vi "ConfigDevice.vi"(8 "error in (no error)":errorcluster, 11 "ChromaAcLoad in":refnum<class "ChromaAcLoad.lvclass">) -> (0 "error out":errorcluster, 3 "ChromaAcLoad out":refnum<class "ChromaAcLoad.lvclass">)   [LabVIEW 2018, in "AcPwrPlugins.lvlib" / "ChromaAcLoad.lvclass"]
doc: "This VI configures the instrument based on the INI file settings or changes to these settings made using the PrefDialog.vi."
uses:
  ChromaAcLoad.lvclass
  C:/Users/ico/Documents/Projects/NistPluggableModules/AcPwr/AcPwrPlugins/AcPwrBaseClass/AcPwrBase.lvclass
  AcPwrBaseClass/AcPwrBase.lvclass/AcPwrBase.ctl
  TypeDefs/RangeCheck.ctl
  AcPwrBaseClass/Accessors/Read BaseConfig.vi
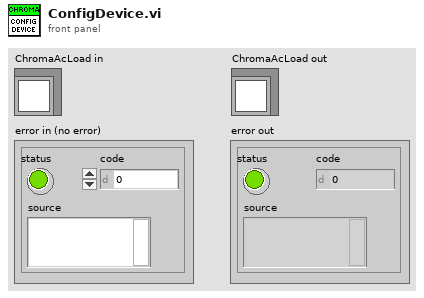
[diagram p1: front panel]
types:
  T1 = typedef "AcPwrPlugins.lvlib/AcPwrBase.lvclass/BaseConfig.ctl" = cluster{"Frequency":dbl, "FrequencyRange":dbl[], "Phases":T2[], "Name":string, "Chroma":T3, "NHRDC":T4, "PPS":T5}
  T2 = typedef "AcPwrPlugins.lvlib/AcPwrBase.lvclass/Phase.ctl" = cluster{"Name":string, "Enabled":bool, "VoltageLevel":dbl, "Handle":string, "VoltageRange":dbl[], "Connected":bool, "CurrentLimit":dbl, "Waveform":string}
  T3 = typedef "AcPwrPlugins.lvlib/ChromaAcLoad.lvclass/DeviceProperties.ctl" = cluster{"Configuration Mode":enum16{"Constant Voltage (DC)", "Constant Power (DC)", "Constant Power (AC)", "Constant Current (DC)", "Constant Current (AC)", "Constant Resistance (DC)", "Constant Resistance (AC)", "Rectified Mode (DC)", "Inrush (AC)", "RLC CP (AC)", "RLC (AC)"}, "Phases":cluster{"Handle":string, "Name":string, "Phase Select":i32, "Instrument Options":string, "id query (T)":bool, "reset device (T)":bool, "Load Short Circuited":bool, "Line Synchronization":bool, "Load Current (A/Arms)":dbl, "Load Voltage (V/Vrms)":dbl, "Load Power (W)":dbl, "Load Resistance (Ohms)":dbl, "Load Current Peak Limit (A)":dbl, "Load Current Limit (A/Arms)":dbl, "Load Power Limit (W)":dbl, "Synch Frequency (Hz)":dbl, "Priority":enum16{"CF Only", "PF Only", "Both (CF)", "Both (PF)"}, "Crest Factor":dbl, "Power Factor":dbl, "Slew Rate":cluster{"Rise Slew Rate (A/ms)":i32, "Fall Slew Rate (A/ms)":i32}, "LC/RLC Mode":cluster{"Capacitance (uF)":i32, "Inductance (uH)":i32, "Series Resistance (Ohm)":dbl, "Parallel Resistance (Ohm)":dbl}, "Timing":cluster{"TimingOn":enum16{""}, "Hours":u32, "Minutes":u32, "Seconds":dbl, "CutoffVoltage":dbl}, "Connected":bool}[]}
  T4 = typedef "AcPwrPlugins.lvlib/NHRDCPower.lvclass/Device(s)Settings.ctl" = cluster{"Handle":string, "Name":string, "id query (Yes)":bool, "reset device (Yes)":bool, "Connected":bool, "Voltage Range (V)":dbl[], "Timing":cluster{"TimingOn":enum16{""}, "Hours":u32, "Minutes":u32, "Seconds":dbl, "CutoffVoltage":dbl}, "Initial Battery Detect Voltage (0)":sgl, "SafetySettings":cluster{"SetWatchDog":bool, "Voltage (V)":sgl, "Current (A)":sgl, "Power (W)":sgl, "Voltage Delay (s)":sgl, "Current Delay (s)":sgl, "Power Delay (s)":sgl}, "Options String":string, "Aperture Time (s)":sgl, "operating state (Off)":i32, "OutputSettings":cluster{"Voltage (V)":sgl, "Current (A)":sgl, "Resistance (Ohms)":sgl, "Power (W)":sgl, "Enable Voltage":bool, "Enable Current":bool, "Enable Resistance":bool, "Enable Power":bool, "Delay After (s)":sgl, "Wait Value (V, A, W)":sgl, "Enable Wait":bool, "Wait on Value":i32}[], "SlewRate":cluster{"Set Voltage Rate V/S":sgl, "Set Current Rate A/S":sgl, "Set Resistance Rate R/S":sgl, "Set Power Rate W/S":sgl}}[]
  T5 = typedef "AcPwrPlugins.lvlib/PacificPowerSource.lvclass/DeviceSettings.ctl" = cluster{"Handle":string, "Connected":bool, "Clear Device (F)":bool, "btnIdQuery":bool, "btnReset":bool, "Program #":cluster{"Phase B (Degrees)":i32, "Waveform A (1: Sine)":i32, "Voltage Level (Va)":dbl, "Program Number (0)":i32, "Voltage Level (Vb) ":dbl, "Form (3: Three)":u16, "Coupling  (0: Direct)":u16, "Frequency (45Hz)":dbl, "Current Limit (40A)":dbl, "Phase C (Degrees)":i32, "Voltage Level (Vc)":dbl, "Waveform B (1: Sine)":i32, "Waveform C (1: Sine)":i32}[], "Impedance Parameters (off, 0.00)":cluster{"State":bool, "Impedance":dbl}, "Transient Execution (F)":bool, "OutputEnabled":bool, "Source Range":cluster{"Frequency Minimum (45 Hz)":dbl, "Frequency Maximum (1200 Hz)":dbl, "Voltage Maximum (V)":dbl, "Voltage Minimum (V)":dbl, "Range Control (0: Auto)":u16, "Initial Voltage (0V)":u16, "Frequency Range (600Hz)":u16}, "Port Type":enum16{"GPIB", "Serial"}}[]
  T6 = enum16{"Constant Voltage (DC)", "Constant Power (DC)", "Constant Power (AC)", "Constant Current (DC)", "Constant Current (AC)", "Constant Resistance (DC)", "Constant Resistance (AC)", "Rectified Mode (DC)", "Inrush (AC)", "RLC CP (AC)", "RLC (AC)"}
  T7 = cluster{"Handle":string, "Name":string, "Phase Select":i32, "Instrument Options":string, "id query (T)":bool, "reset device (T)":bool, "Load Short Circuited":bool, "Line Synchronization":bool, "Load Current (A/Arms)":dbl, "Load Voltage (V/Vrms)":dbl, "Load Power (W)":dbl, "Load Resistance (Ohms)":dbl, "Load Current Peak Limit (A)":dbl, "Load Current Limit (A/Arms)":dbl, "Load Power Limit (W)":dbl, "Synch Frequency (Hz)":dbl, "Priority":enum16{"CF Only", "PF Only", "Both (CF)", "Both (PF)"}, "Crest Factor":dbl, "Power Factor":dbl, "Slew Rate":cluster{"Rise Slew Rate (A/ms)":i32, "Fall Slew Rate (A/ms)":i32}, "LC/RLC Mode":cluster{"Capacitance (uF)":i32, "Inductance (uH)":i32, "Series Resistance (Ohm)":dbl, "Parallel Resistance (Ohm)":dbl}, "Timing":cluster{"TimingOn":enum16{""}, "Hours":u32, "Minutes":u32, "Seconds":dbl, "CutoffVoltage":dbl}, "Connected":bool}[]
  T8 = typedef "AcPwrPlugins.lvlib/ChromaAcLoad.lvclass/RangeCheck.ctl" = enum16{"Power", "Power Limit", "Current", "Current Peak", "Current Limit", "Voltage", "AC Resistance", "DC Resistance", "Frequency", "Crest Factor", "Power Factor", "RLC Power Factor", "Rise Slew Rate", "Fall Slew Rate", "Capacitance", "Inductance", "Parallel Resistance", "Series Resistance"}[]
  T9 = enum16{"CF Only", "PF Only", "Both (CF)", "Both (PF)"}
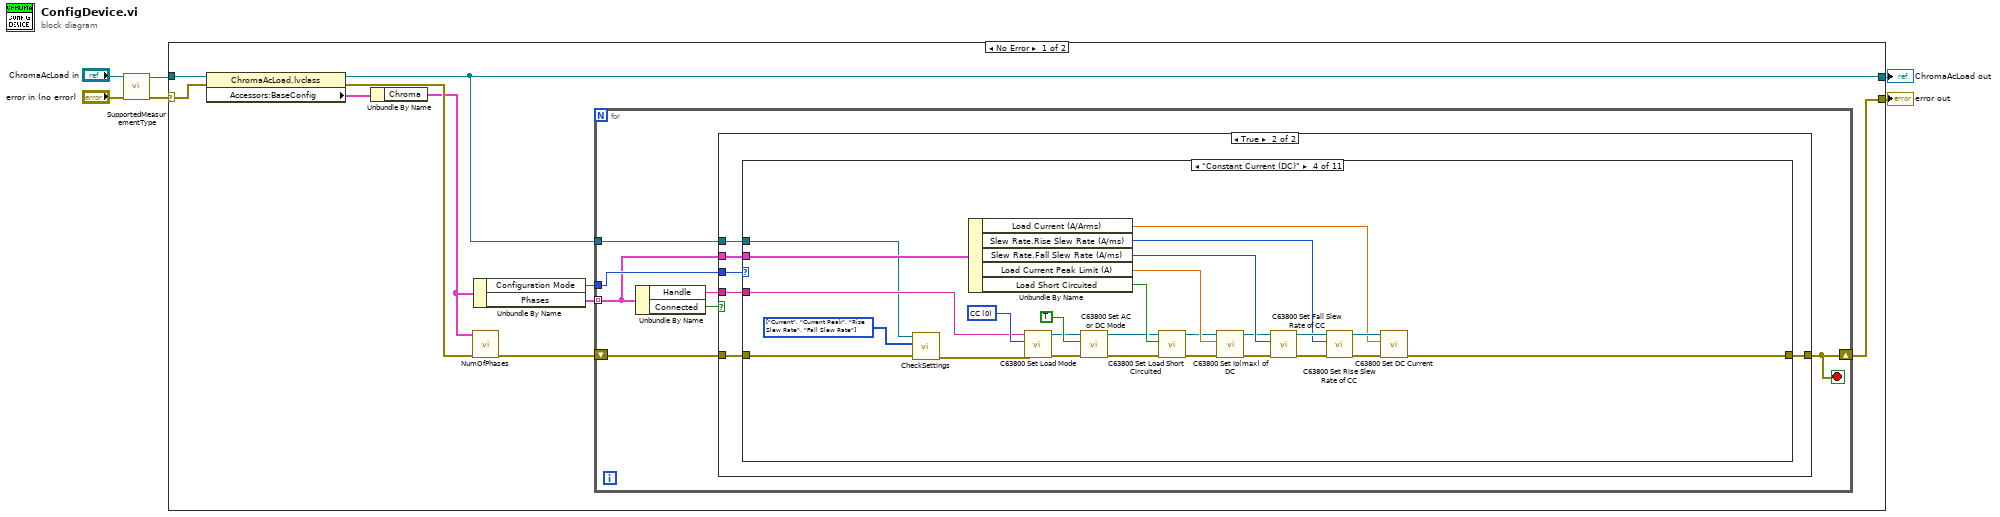
[diagram p0: block diagram]
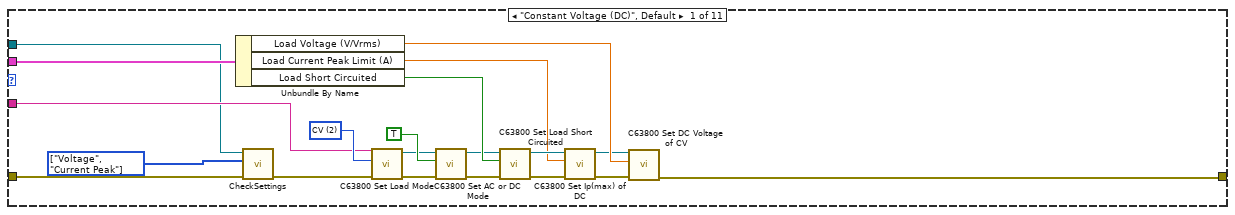
[diagram p3: hidden frame]
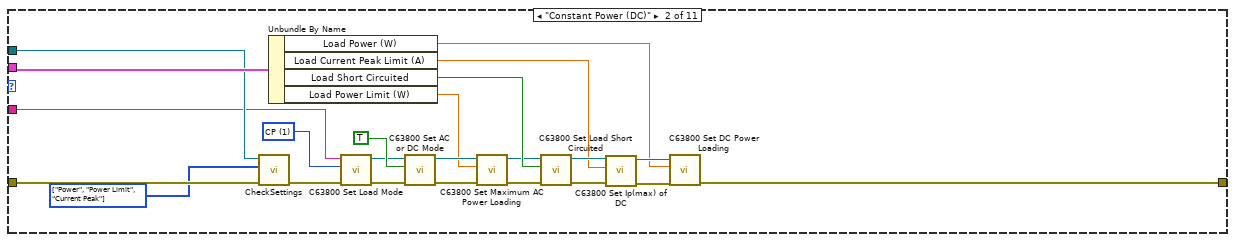
[diagram p4: hidden frame]
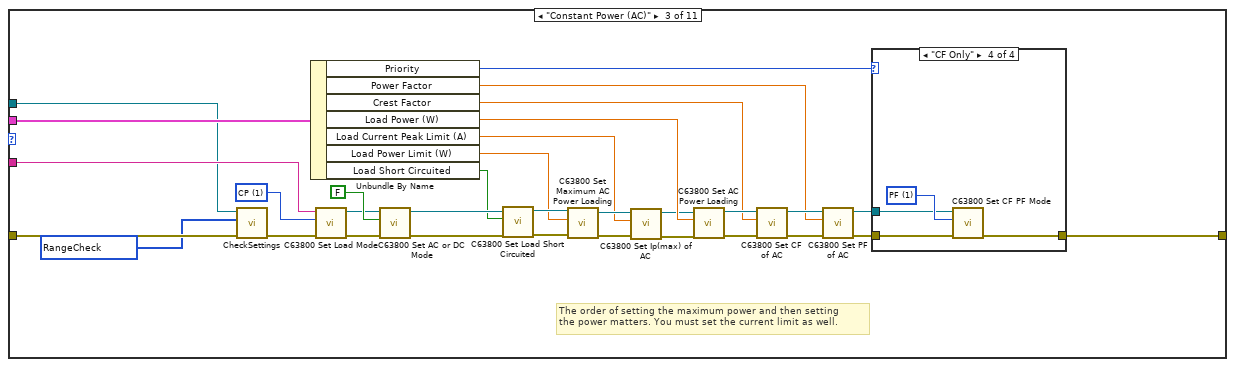
[diagram p5: hidden frame]
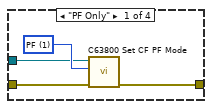
[diagram p6: hidden frame]
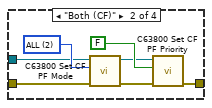
[diagram p7: hidden frame]
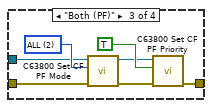
[diagram p8: hidden frame]
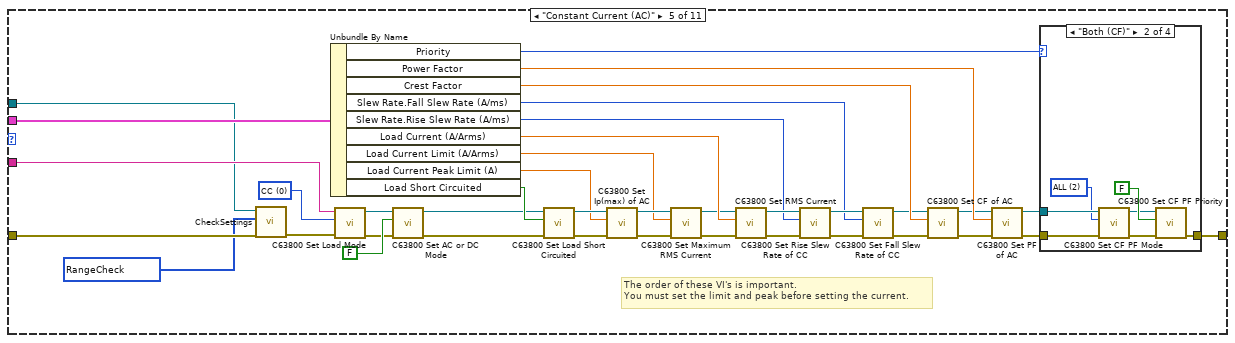
[diagram p9: hidden frame]
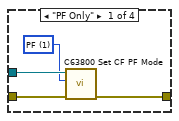
[diagram p10: hidden frame]
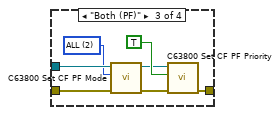
[diagram p11: hidden frame]
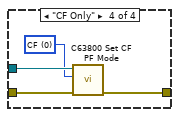
[diagram p12: hidden frame]
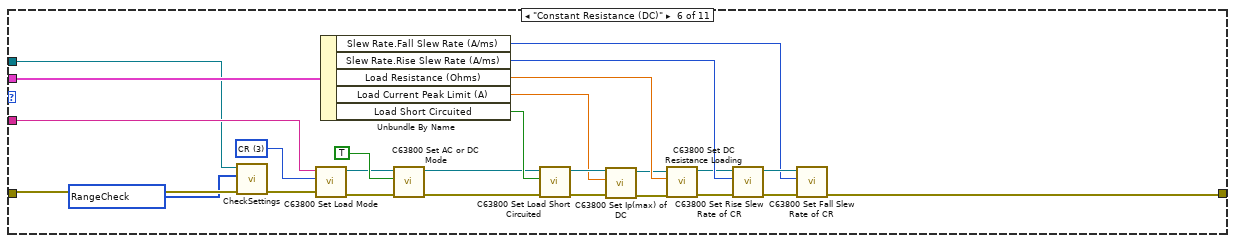
[diagram p13: hidden frame]
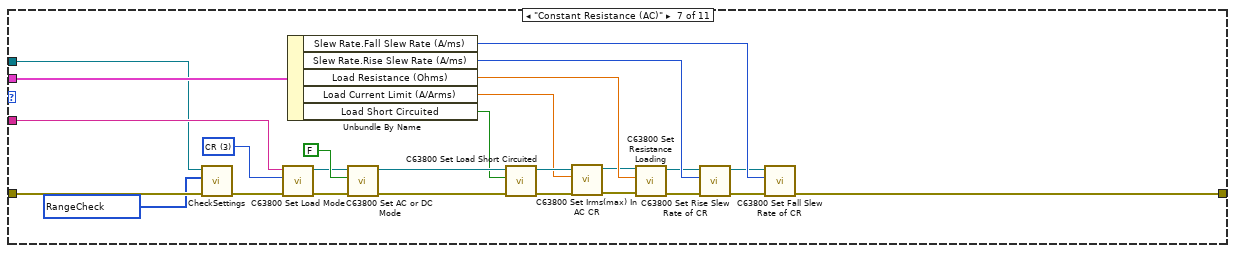
[diagram p14: hidden frame]
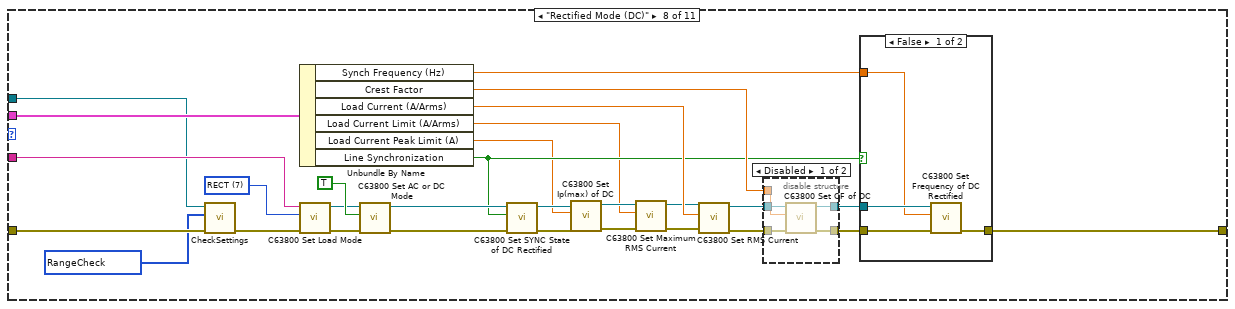
[diagram p15: hidden frame]
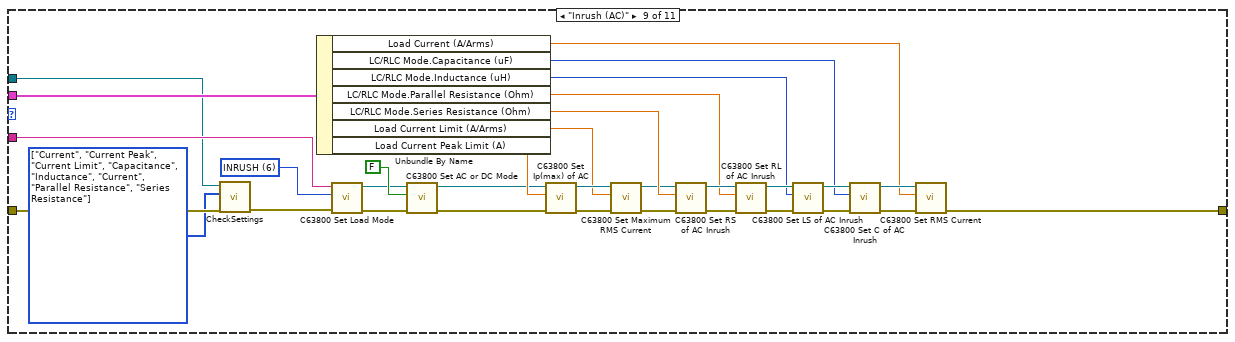
[diagram p18: hidden frame]
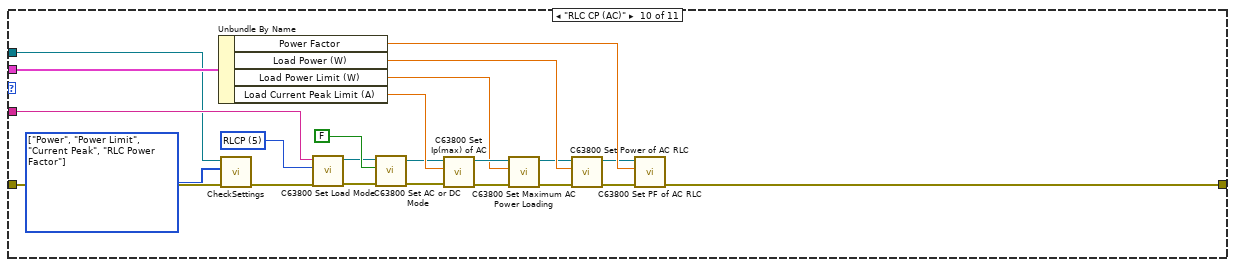
[diagram p19: hidden frame]
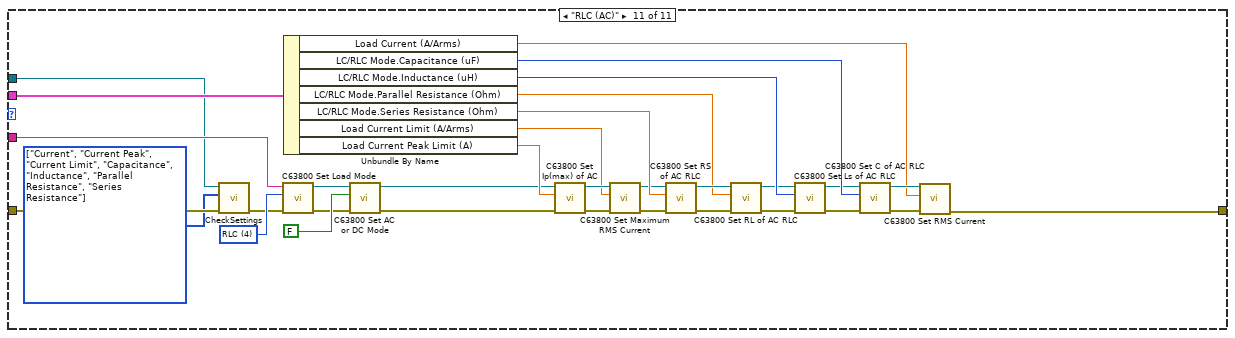
[diagram p20: hidden frame]
diagram:
  n1 = call-dynamic "SupportedMeasurementType.vi"("error in (no error)"="error in (no error)", "ChromaAcLoad in"="ChromaAcLoad in") -> ("error out"=w3:errorcluster, "ChromaAcLoad out"=w4:refnum<class "ChromaAcLoad.lvclass">)  [unwired: 8 in]
  n2 = case shown="No Error" w3 {
    selector: w3 -> [w16 w391]
    tunnel: [w15 w391] -> w6
    tunnel: w4 -> [w14 w390]
    tunnel: [w13 w390] -> w5
    frame No Error {
      n3 = property class="ChromaAcLoad.lvclass"(reference=w14, error in=w16) -> (reference out=w13:refnum<class "ChromaAcLoad.lvclass">, error out=w9:errorcluster, "Accessors:BaseConfig"=w8:T1)
      n4 = Unbundle By Name(w8) -> ("Chroma"=w7:T3)
      n5 = call "NumOfPhases.vi"("Error In"=w9, "Device Properties"=w7) -> ("Error Out"=w10:errorcluster)  [unwired: 8 in, 1 out]
      n6 = Unbundle By Name(w7) -> ("Configuration Mode"=w11:T6, "Phases"=w12:T7)
      n7 = for {
        shift-right: [w20] -> w15
        shift-left: w10 -> [w21]
        tunnel: w12 -> [w18] mode=indexing
        tunnel: w11 -> [w23]
        tunnel: w13 -> [w17]
        stop <- w20 stop-if-true
        n8 = Unbundle By Name(w18) -> ("Handle"=w19:string, "Connected"=w22:bool)
        n9 = case shown="True" w22 {
          tunnel: w23 -> [_ w28]
          tunnel: w21 -> [w24 w30]
          tunnel: [w24 w29] -> w20
          tunnel: w19 -> [_ w27]
          tunnel: w18 -> [_ w26]
          tunnel: w17 -> [_ w25]
          frame False {
          }
          frame True {
            n10 = case shown="\"Constant Current (DC)\"" w28 {
              tunnel: w30 -> [w39 w71 w102 w137 w167 w218 w252 w278 w314 w347 w371]
              tunnel: [w41 w69 w105 w128 w178 w228 w261 w286 w310 w342 w364] -> w29
              tunnel: w27 -> [w43 w70 w103 w140 w173 w221 w255 w279 w316 w349 w373]
              tunnel: w26 -> [w49 w73 w104 w146 w179 w226 w260 w285 w323 w356 w378]
              tunnel: w25 -> [w37 w72 w101 w136 w166 w216 w250 w276 w315 w345 w368]
              frame "Constant Voltage (DC)", Default {
                w36 = T8 [enum."Voltage", enum."Current Peak"] items=["Power", "Power Limit", "Current", "Current Peak", "Current Limit", "Voltage", "AC Resistance", "DC Resistance", "Frequency", "Crest Factor", "Power Factor", "RLC Power Factor", "Rise Slew Rate", "Fall Slew Rate", "Capacitance", "Inductance", "Parallel Resistance", "Series Resistance"] ("RangeCheck")
                w45 = 2 items=["CC", "CP", "CV", "CR", "RLC", "RLCP", "INRUSH", "RECT"] ("Load Mode")
                n11 = Unbundle By Name(w49) -> ("Load Voltage (V/Vrms)"=w40:dbl, "Load Current Peak Limit (A)"=w31:dbl, "Load Short Circuited"=w50:bool)
                n12 = call-dynamic "CheckSettings.vi"("ChromaAcLoad in"=w37, "RangeCheck"=w36, "error in (no error)"=w39) -> ("error out"=w38:errorcluster)  [unwired: 6 in, 1 out]
                n13 = call <instrlib>:"C63800 Set Load Mode.vi"("error in (no error)"=w38, "Load Mode"=w45, "Instrument Handle"=w43) -> ("error out"=w44:errorcluster, "Instrument Handle out"=w42:refnum<k15>)  [unwired: 7 in]
                n14 = call <instrlib>:"C63800 Set AC or DC Mode.vi"("error in (no error)"=w44, "Select AC_DC Mode"=TRUE, "Instrument Handle"=w42) -> ("error out"=w48:errorcluster, "Instrument Handle out"=w46:refnum<k15>)  [unwired: 7 in]
                n15 = call <instrlib>:"C63800 Set Load Short Circuited.vi"("error in (no error)"=w48, "Short Circuited State"=w50, "Instrument Handle"=w46) -> ("error out"=w35:errorcluster, "Instrument Handle out"=w32:refnum<k15>)  [unwired: 7 in]
                n16 = call <instrlib>:"C63800 Set Ip(max) of DC.vi"("error in (no error)"=w35, "I_max_DC"=w31, "Instrument Handle"=w32) -> ("error out"=w33:errorcluster, "Instrument Handle out"=w34:refnum<k15>)  [unwired: 7 in]
                n17 = call <instrlib>:"C63800 Set DC Voltage of CV.vi"("error in (no error)"=w33, "SetDCVoltageofCV"=w40, "Instrument Handle"=w34) -> ("error out"=w41:errorcluster)  [unwired: 7 in, 1 out]
              }
              frame "Constant Power (DC)" {
                w60 = T8 [enum."Power", enum."Power Limit", enum."Current Peak"] items=["Power", "Power Limit", "Current", "Current Peak", "Current Limit", "Voltage", "AC Resistance", "DC Resistance", "Frequency", "Crest Factor", "Power Factor", "RLC Power Factor", "Rise Slew Rate", "Fall Slew Rate", "Capacitance", "Inductance", "Parallel Resistance", "Series Resistance"] ("RangeCheck")
                w66 = 1 items=["CC", "CP", "CV", "CR", "RLC", "RLCP", "INRUSH", "RECT"] ("Load Mode")
                n18 = call-dynamic "CheckSettings.vi"("ChromaAcLoad in"=w72, "RangeCheck"=w60, "error in (no error)"=w71) -> ("error out"=w63:errorcluster)  [unwired: 6 in, 1 out]
                n19 = Unbundle By Name(w73) -> ("Load Power (W)"=w55:dbl, "Load Current Peak Limit (A)"=w54:dbl, "Load Short Circuited"=w68:bool, "Load Power Limit (W)"=w51:dbl)
                n20 = call <instrlib>:"C63800 Set Load Mode.vi"("error in (no error)"=w63, "Load Mode"=w66, "Instrument Handle"=w70) -> ("error out"=w65:errorcluster, "Instrument Handle out"=w64:refnum<k15>)  [unwired: 7 in]
                n21 = call <instrlib>:"C63800 Set AC or DC Mode.vi"("error in (no error)"=w65, "Select AC_DC Mode"=TRUE, "Instrument Handle"=w64) -> ("error out"=w52:errorcluster, "Instrument Handle out"=w53:refnum<k15>)  [unwired: 7 in]
                n22 = call <instrlib>:"C63800 Set Maximum AC Power Loading.vi"("error in (no error)"=w52, "AC Maximum Power Loading"=w51, "Instrument Handle"=w53) -> ("error out"=w62:errorcluster, "Instrument Handle out"=w61:refnum<k15>)  [unwired: 7 in]
                n23 = call <instrlib>:"C63800 Set Load Short Circuited.vi"("error in (no error)"=w62, "Short Circuited State"=w68, "Instrument Handle"=w61) -> ("error out"=w59:errorcluster, "Instrument Handle out"=w56:refnum<k15>)  [unwired: 7 in]
                n24 = call <instrlib>:"C63800 Set Ip(max) of DC.vi"("error in (no error)"=w59, "I_max_DC"=w54, "Instrument Handle"=w56) -> ("error out"=w58:errorcluster, "Instrument Handle out"=w57:refnum<k15>)  [unwired: 7 in]
                n25 = call <instrlib>:"C63800 Set DC Power Loading.vi"("error in (no error)"=w58, "DC Power Loading"=w55, "Instrument Handle"=w57) -> ("error out"=w69:errorcluster)  [unwired: 7 in, 1 out]
              }
              frame "Constant Power (AC)" {
                w93 = T8 [enum."Power", enum."Power Limit", enum."Current Peak", enum."Power Factor", enum."Crest Factor"] items=["Power", "Power Limit", "Current", "Current Peak", "Current Limit", "Voltage", "AC Resistance", "DC Resistance", "Frequency", "Crest Factor", "Power Factor", "RLC Power Factor", "Rise Slew Rate", "Fall Slew Rate", "Capacitance", "Inductance", "Parallel Resistance", "Series Resistance"] ("RangeCheck")
                w97 = 1 items=["CC", "CP", "CV", "CR", "RLC", "RLCP", "INRUSH", "RECT"] ("Load Mode")
                # "The order of setting the maximum power and then setting \nthe power matters. You must set the current limit as well."
                n26 = call-dynamic "CheckSettings.vi"("ChromaAcLoad in"=w101, "RangeCheck"=w93, "error in (no error)"=w102) -> ("error out"=w94:errorcluster)  [unwired: 6 in, 1 out]
                n27 = Unbundle By Name(w104) -> ("Priority"=w90:T9, "Power Factor"=w82:dbl, "Crest Factor"=w83:dbl, "Load Power (W)"=w92:dbl, "Load Current Peak Limit (A)"=w77:dbl, "Load Power Limit (W)"=w74:dbl, "Load Short Circuited"=w91:bool)
                n28 = call <instrlib>:"C63800 Set Load Mode.vi"("error in (no error)"=w94, "Load Mode"=w97, "Instrument Handle"=w103) -> ("error out"=w96:errorcluster, "Instrument Handle out"=w95:refnum<k15>)  [unwired: 7 in]
                n29 = call <instrlib>:"C63800 Set AC or DC Mode.vi"("error in (no error)"=w96, "Select AC_DC Mode"=FALSE, "Instrument Handle"=w95) -> ("error out"=w100:errorcluster, "Instrument Handle out"=w99:refnum<k15>)  [unwired: 7 in]
                n30 = call <instrlib>:"C63800 Set Load Short Circuited.vi"("error in (no error)"=w100, "Short Circuited State"=w91, "Instrument Handle"=w99) -> ("error out"=w75:errorcluster, "Instrument Handle out"=w76:refnum<k15>)  [unwired: 7 in]
                n31 = call <instrlib>:"C63800 Set Maximum AC Power Loading.vi"("error in (no error)"=w75, "AC Maximum Power Loading"=w74, "Instrument Handle"=w76) -> ("error out"=w81:errorcluster, "Instrument Handle out"=w78:refnum<k15>)  [unwired: 7 in]
                n32 = call <instrlib>:"C63800 Set Ip(max) of AC.vi"("error in (no error)"=w81, "Current Peak Max"=w77, "Instrument Handle"=w78) -> ("error out"=w80:errorcluster, "Instrument Handle out"=w79:refnum<k15>)  [unwired: 7 in]
                n33 = call <instrlib>:"C63800 Set AC Power Loading.vi"("error in (no error)"=w80, "AC Power Loading"=w92, "Instrument Handle"=w79) -> ("error out"=w87:errorcluster, "Instrument Handle out"=w86:refnum<k15>)  [unwired: 7 in]
                n34 = call <instrlib>:"C63800 Set CF of AC.vi"("error in (no error)"=w87, "CF of AC"=w83, "Instrument Handle"=w86) -> ("error out"=w89:errorcluster, "Instrument Handle out"=w88:refnum<k15>)  [unwired: 7 in]
                n35 = call <instrlib>:"C63800 Set PF of AC.vi"("error in (no error)"=w89, "PF of AC"=w82, "Instrument Handle"=w88) -> ("error out"=w85:errorcluster, "Instrument Handle out"=w84:refnum<k15>)  [unwired: 7 in]
                n36 = case shown="\"CF Only\"" w90 {
                  tunnel: [w108 w113 w119 w124] -> w105
                  tunnel: w85 -> [w107 w111 w116 w122]
                  tunnel: w84 -> [w106 w110 w117 w123]
                  frame "PF Only" {
                    w109 = 1 items=["CF", "PF", "ALL"] ("CF_PF Mode")
                    n37 = call <instrlib>:"C63800 Set CF PF Mode.vi"("error in (no error)"=w107, "CF_PF Mode"=w109, "Instrument Handle"=w106) -> ("error out"=w108:errorcluster)  [unwired: 7 in, 1 out]
                  }
                  frame "Both (CF)" {
                    w115 = 2 items=["CF", "PF", "ALL"] ("CF_PF Mode")
                    n38 = call <instrlib>:"C63800 Set CF PF Mode.vi"("error in (no error)"=w111, "CF_PF Mode"=w115, "Instrument Handle"=w110) -> ("error out"=w113:errorcluster, "Instrument Handle out"=w112:refnum<k15>)  [unwired: 7 in]
                    n39 = call <instrlib>:"C63800 Set CF PF Priority.vi"("error in (no error)"=w113, "Priority"=FALSE, "Instrument Handle"=w112) -> ()  [unwired: 7 in, 2 out]
                  }
                  frame "Both (PF)" {
                    w121 = 2 items=["CF", "PF", "ALL"] ("CF_PF Mode")
                    n40 = call <instrlib>:"C63800 Set CF PF Mode.vi"("error in (no error)"=w116, "CF_PF Mode"=w121, "Instrument Handle"=w117) -> ("error out"=w119:errorcluster, "Instrument Handle out"=w118:refnum<k15>)  [unwired: 7 in]
                    n41 = call <instrlib>:"C63800 Set CF PF Priority.vi"("error in (no error)"=w119, "Priority"=TRUE, "Instrument Handle"=w118) -> ()  [unwired: 7 in, 2 out]
                  }
                  frame "CF Only" {
                    w125 = 1 items=["CF", "PF", "ALL"] ("CF_PF Mode")
                    n42 = call <instrlib>:"C63800 Set CF PF Mode.vi"("error in (no error)"=w122, "CF_PF Mode"=w125, "Instrument Handle"=w123) -> ("error out"=w124:errorcluster)  [unwired: 7 in, 1 out]
                  }
                }
              }
              frame "Constant Current (DC)" {
                w126 = T8 [enum."Current", enum."Current Peak", enum."Rise Slew Rate", enum."Fall Slew Rate"] items=["Power", "Power Limit", "Current", "Current Peak", "Current Limit", "Voltage", "AC Resistance", "DC Resistance", "Frequency", "Crest Factor", "Power Factor", "RLC Power Factor", "Rise Slew Rate", "Fall Slew Rate", "Capacitance", "Inductance", "Parallel Resistance", "Series Resistance"] ("RangeCheck")
                w143 = 0 items=["CC", "CP", "CV", "CR", "RLC", "RLCP", "INRUSH", "RECT"] ("Load Mode")
                n43 = call-dynamic "CheckSettings.vi"("ChromaAcLoad in"=w136, "RangeCheck"=w126, "error in (no error)"=w137) -> ("error out"=w138:errorcluster)  [unwired: 6 in, 1 out]
                n44 = Unbundle By Name(w146) -> ("Load Current (A/Arms)"=w127:dbl, "Slew Rate.Rise Slew Rate (A/ms)"=w148:i32, "Slew Rate.Fall Slew Rate (A/ms)"=w149:i32, "Load Current Peak Limit (A)"=w132:dbl, "Load Short Circuited"=w147:bool)
                n45 = call <instrlib>:"C63800 Set Load Mode.vi"("error in (no error)"=w138, "Load Mode"=w143, "Instrument Handle"=w140) -> ("error out"=w142:errorcluster, "Instrument Handle out"=w141:refnum<k15>)  [unwired: 7 in]
                n46 = call <instrlib>:"C63800 Set AC or DC Mode.vi"("error in (no error)"=w142, "Select AC_DC Mode"=TRUE, "Instrument Handle"=w141) -> ("error out"=w139:errorcluster, "Instrument Handle out"=w144:refnum<k15>)  [unwired: 7 in]
                n47 = call <instrlib>:"C63800 Set Load Short Circuited.vi"("error in (no error)"=w139, "Short Circuited State"=w147, "Instrument Handle"=w144) -> ("error out"=w135:errorcluster, "Instrument Handle out"=w131:refnum<k15>)  [unwired: 7 in]
                n48 = call <instrlib>:"C63800 Set Ip(max) of DC.vi"("error in (no error)"=w135, "I_max_DC"=w132, "Instrument Handle"=w131) -> ("error out"=w134:errorcluster, "Instrument Handle out"=w133:refnum<k15>)  [unwired: 7 in]
                n49 = call <instrlib>:"C63800 Set Fall Slew Rate of CC.vi"("error in (no error)"=w134, "Fall Slew Rate of CC"=w149, "Instrument Handle"=w133) -> ("error out"=w151:errorcluster, "Instrument Handle out"=w150:refnum<k15>)  [unwired: 7 in]
                n50 = call <instrlib>:"C63800 Set Rise Slew Rate of CC.vi"("error in (no error)"=w151, "Rise Slew Rate of CC"=w148, "Instrument Handle"=w150) -> ("error out"=w130:errorcluster, "Instrument Handle out"=w129:refnum<k15>)  [unwired: 7 in]
                n51 = call <instrlib>:"C63800 Set DC Current.vi"("error in (no error)"=w130, "Set DC Current"=w127, "Instrument Handle"=w129) -> ("error out"=w128:errorcluster)  [unwired: 7 in, 1 out]
              }
              frame "Constant Current (AC)" {
                w165 = T8 [enum."Current", enum."Current Peak", enum."Current Limit", enum."Power Factor", enum."Crest Factor", enum."Fall Slew Rate", enum."Rise Slew Rate"] items=["Power", "Power Limit", "Current", "Current Peak", "Current Limit", "Voltage", "AC Resistance", "DC Resistance", "Frequency", "Crest Factor", "Power Factor", "RLC Power Factor", "Rise Slew Rate", "Fall Slew Rate", "Capacitance", "Inductance", "Parallel Resistance", "Series Resistance"] ("RangeCheck")
                w175 = 0 items=["CC", "CP", "CV", "CR", "RLC", "RLCP", "INRUSH", "RECT"] ("Load Mode")
                # "The order of these VI's is important. \nYou must set the limit and peak before setting the current."
                n52 = call-dynamic "CheckSettings.vi"("ChromaAcLoad in"=w166, "RangeCheck"=w165, "error in (no error)"=w167) -> ("error out"=w168:errorcluster)  [unwired: 6 in, 1 out]
                n53 = Unbundle By Name(w179) -> ("Priority"=w185:T9, "Power Factor"=w188:dbl, "Crest Factor"=w187:dbl, "Slew Rate.Fall Slew Rate (A/ms)"=w157:i32, "Slew Rate.Rise Slew Rate (A/ms)"=w158:i32, "Load Current (A/Arms)"=w170:dbl, "Load Current Limit (A/Arms)"=w152:dbl, "Load Current Peak Limit (A)"=w153:dbl, "Load Short Circuited"=w180:bool)
                n54 = call <instrlib>:"C63800 Set Load Mode.vi"("error in (no error)"=w168, "Load Mode"=w175, "Instrument Handle"=w173) -> ("error out"=w174:errorcluster, "Instrument Handle out"=w172:refnum<k15>)  [unwired: 7 in]
                n55 = call <instrlib>:"C63800 Set AC or DC Mode.vi"("error in (no error)"=w174, "Select AC_DC Mode"=FALSE, "Instrument Handle"=w172) -> ("error out"=w169:errorcluster, "Instrument Handle out"=w176:refnum<k15>)  [unwired: 7 in]
                n56 = call <instrlib>:"C63800 Set Load Short Circuited.vi"("error in (no error)"=w169, "Short Circuited State"=w180, "Instrument Handle"=w176) -> ("error out"=w181:errorcluster, "Instrument Handle out"=w182:refnum<k15>)  [unwired: 7 in]
                n57 = call <instrlib>:"C63800 Set Ip(max) of AC.vi"("error in (no error)"=w181, "Current Peak Max"=w153, "Instrument Handle"=w182) -> ("error out"=w171:errorcluster, "Instrument Handle out"=w155:refnum<k15>)  [unwired: 7 in]
                n58 = call <instrlib>:"C63800 Set Maximum RMS Current.vi"("error in (no error)"=w171, "Set Max RMS Current"=w152, "Instrument Handle"=w155) -> ("error out"=w156:errorcluster, "Instrument Handle out"=w154:refnum<k15>)  [unwired: 7 in]
                n59 = call <instrlib>:"C63800 Set RMS Current.vi"("error in (no error)"=w156, "Set RMS Current"=w170, "Instrument Handle"=w154) -> ("error out"=w164:errorcluster, "Instrument Handle out"=w163:refnum<k15>)  [unwired: 7 in]
                n60 = call <instrlib>:"C63800 Set Rise Slew Rate of CC.vi"("error in (no error)"=w164, "Rise Slew Rate of CC"=w158, "Instrument Handle"=w163) -> ("error out"=w162:errorcluster, "Instrument Handle out"=w161:refnum<k15>)  [unwired: 7 in]
                n61 = call <instrlib>:"C63800 Set Fall Slew Rate of CC.vi"("error in (no error)"=w162, "Fall Slew Rate of CC"=w157, "Instrument Handle"=w161) -> ("error out"=w159:errorcluster, "Instrument Handle out"=w160:refnum<k15>)  [unwired: 7 in]
                n62 = call <instrlib>:"C63800 Set CF of AC.vi"("error in (no error)"=w159, "CF of AC"=w187, "Instrument Handle"=w160) -> ("error out"=w189:errorcluster, "Instrument Handle out"=w186:refnum<k15>)  [unwired: 7 in]
                n63 = call <instrlib>:"C63800 Set PF of AC.vi"("error in (no error)"=w189, "PF of AC"=w188, "Instrument Handle"=w186) -> ("error out"=w183:errorcluster, "Instrument Handle out"=w184:refnum<k15>)  [unwired: 7 in]
                n64 = case shown="\"Both (CF)\"" w185 {
                  tunnel: w184 -> [w193 w199 w205 w209]
                  tunnel: w183 -> [w192 w198 w204 w208]
                  tunnel: [w190 w195 w201 w206] -> w178
                  frame "PF Only" {
                    w191 = 1 items=["CF", "PF", "ALL"] ("CF_PF Mode")
                    n65 = call <instrlib>:"C63800 Set CF PF Mode.vi"("error in (no error)"=w192, "CF_PF Mode"=w191, "Instrument Handle"=w193) -> ("error out"=w190:errorcluster)  [unwired: 7 in, 1 out]
                  }
                  frame "Both (CF)" {
                    w197 = 2 items=["CF", "PF", "ALL"] ("CF_PF Mode")
                    n66 = call <instrlib>:"C63800 Set CF PF Mode.vi"("error in (no error)"=w198, "CF_PF Mode"=w197, "Instrument Handle"=w199) -> ("error out"=w195:errorcluster, "Instrument Handle out"=w194:refnum<k15>)  [unwired: 7 in]
                    n67 = call <instrlib>:"C63800 Set CF PF Priority.vi"("error in (no error)"=w195, "Priority"=FALSE, "Instrument Handle"=w194) -> ()  [unwired: 7 in, 2 out]
                  }
                  frame "Both (PF)" {
                    w203 = 2 items=["CF", "PF", "ALL"] ("CF_PF Mode")
                    n68 = call <instrlib>:"C63800 Set CF PF Mode.vi"("error in (no error)"=w204, "CF_PF Mode"=w203, "Instrument Handle"=w205) -> ("error out"=w201:errorcluster, "Instrument Handle out"=w200:refnum<k15>)  [unwired: 7 in]
                    n69 = call <instrlib>:"C63800 Set CF PF Priority.vi"("error in (no error)"=w201, "Priority"=TRUE, "Instrument Handle"=w200) -> ()  [unwired: 7 in, 2 out]
                  }
                  frame "CF Only" {
                    w207 = 0 items=["CF", "PF", "ALL"] ("CF_PF Mode")
                    n70 = call <instrlib>:"C63800 Set CF PF Mode.vi"("error in (no error)"=w208, "CF_PF Mode"=w207, "Instrument Handle"=w209) -> ("error out"=w206:errorcluster)  [unwired: 7 in, 1 out]
                  }
                }
              }
              frame "Constant Resistance (DC)" {
                w215 = T8 [enum."DC Resistance", enum."Current Peak", enum."Rise Slew Rate", enum."Fall Slew Rate"] items=["Power", "Power Limit", "Current", "Current Peak", "Current Limit", "Voltage", "AC Resistance", "DC Resistance", "Frequency", "Crest Factor", "Power Factor", "RLC Power Factor", "Rise Slew Rate", "Fall Slew Rate", "Capacitance", "Inductance", "Parallel Resistance", "Series Resistance"] ("RangeCheck")
                w223 = 3 items=["CC", "CP", "CV", "CR", "RLC", "RLCP", "INRUSH", "RECT"] ("Load Mode")
                n71 = call-dynamic "CheckSettings.vi"("ChromaAcLoad in"=w216, "RangeCheck"=w215, "error in (no error)"=w218) -> ("error out"=w217:errorcluster)  [unwired: 6 in, 1 out]
                n72 = call <instrlib>:"C63800 Set Load Mode.vi"("error in (no error)"=w217, "Load Mode"=w223, "Instrument Handle"=w221) -> ("error out"=w222:errorcluster, "Instrument Handle out"=w220:refnum<k15>)  [unwired: 7 in]
                n73 = Unbundle By Name(w226) -> ("Slew Rate.Fall Slew Rate (A/ms)"=w232:i32, "Slew Rate.Rise Slew Rate (A/ms)"=w231:i32, "Load Resistance (Ohms)"=w235:dbl, "Load Current Peak Limit (A)"=w210:dbl, "Load Short Circuited"=w227:bool)
                n74 = call <instrlib>:"C63800 Set AC or DC Mode.vi"("error in (no error)"=w222, "Select AC_DC Mode"=TRUE, "Instrument Handle"=w220) -> ("error out"=w219:errorcluster, "Instrument Handle out"=w225:refnum<k15>)  [unwired: 7 in]
                n75 = call <instrlib>:"C63800 Set Load Short Circuited.vi"("error in (no error)"=w219, "Short Circuited State"=w227, "Instrument Handle"=w225) -> ("error out"=w212:errorcluster, "Instrument Handle out"=w211:refnum<k15>)  [unwired: 7 in]
                n76 = call <instrlib>:"C63800 Set Ip(max) of DC.vi"("error in (no error)"=w212, "I_max_DC"=w210, "Instrument Handle"=w211) -> ("error out"=w214:errorcluster, "Instrument Handle out"=w213:refnum<k15>)  [unwired: 7 in]
                n77 = call <instrlib>:"C63800 Set DC Resistance Loading.vi"("error in (no error)"=w214, "DC Resistance Loading"=w235, "Instrument Handle"=w213) -> ("error out"=w229:errorcluster, "Instrument Handle out"=w230:refnum<k15>)  [unwired: 7 in]
                n78 = call <instrlib>:"C63800 Set Rise Slew Rate of CR.vi"("error in (no error)"=w229, "Rise Slew Rate of CR"=w231, "Instrument Handle"=w230) -> ("error out"=w233:errorcluster, "Instrument Handle out"=w234:refnum<k15>)  [unwired: 7 in]
                n79 = call <instrlib>:"C63800 Set Fall Slew Rate of CR.vi"("error in (no error)"=w233, "Fall Slew Rate of CR"=w232, "Instrument Handle"=w234) -> ("error out"=w228:errorcluster)  [unwired: 7 in, 1 out]
              }
              frame "Constant Resistance (AC)" {
                w249 = T8 [enum."AC Resistance", enum."Current Limit", enum."Rise Slew Rate", enum."Fall Slew Rate"] items=["Power", "Power Limit", "Current", "Current Peak", "Current Limit", "Voltage", "AC Resistance", "DC Resistance", "Frequency", "Crest Factor", "Power Factor", "RLC Power Factor", "Rise Slew Rate", "Fall Slew Rate", "Capacitance", "Inductance", "Parallel Resistance", "Series Resistance"] ("RangeCheck")
                w257 = 3 items=["CC", "CP", "CV", "CR", "RLC", "RLCP", "INRUSH", "RECT"] ("Load Mode")
                n80 = call-dynamic "CheckSettings.vi"("ChromaAcLoad in"=w250, "RangeCheck"=w249, "error in (no error)"=w252) -> ("error out"=w251:errorcluster)  [unwired: 6 in, 1 out]
                n81 = call <instrlib>:"C63800 Set Load Mode.vi"("error in (no error)"=w251, "Load Mode"=w257, "Instrument Handle"=w255) -> ("error out"=w256:errorcluster, "Instrument Handle out"=w254:refnum<k15>)  [unwired: 7 in]
                n82 = Unbundle By Name(w260) -> ("Slew Rate.Fall Slew Rate (A/ms)"=w242:i32, "Slew Rate.Rise Slew Rate (A/ms)"=w244:i32, "Load Resistance (Ohms)"=w245:dbl, "Load Current Limit (A/Arms)"=w236:dbl, "Load Short Circuited"=w246:bool)
                n83 = call <instrlib>:"C63800 Set AC or DC Mode.vi"("error in (no error)"=w256, "Select AC_DC Mode"=FALSE, "Instrument Handle"=w254) -> ("error out"=w253:errorcluster, "Instrument Handle out"=w259:refnum<k15>)  [unwired: 7 in]
                n84 = call <instrlib>:"C63800 Set Load Short Circuited.vi"("error in (no error)"=w253, "Short Circuited State"=w246, "Instrument Handle"=w259) -> ("error out"=w240:errorcluster, "Instrument Handle out"=w239:refnum<k15>)  [unwired: 7 in]
                n85 = call <instrlib>:"C63800 Set Irms(max) In AC CR.vi"("error in (no error)"=w240, "I_max"=w236, "Instrument Handle"=w239) -> ("error out"=w237:errorcluster, "Instrument Handle out"=w238:refnum<k15>)  [unwired: 7 in]
                n86 = call <instrlib>:"C63800 Set Resistance Loading.vi"("error in (no error)"=w237, "Resistance Loading"=w245, "Instrument Handle"=w238) -> ("error out"=w247:errorcluster, "Instrument Handle out"=w243:refnum<k15>)  [unwired: 7 in]
                n87 = call <instrlib>:"C63800 Set Rise Slew Rate of CR.vi"("error in (no error)"=w247, "Rise Slew Rate of CR"=w244, "Instrument Handle"=w243) -> ("error out"=w248:errorcluster, "Instrument Handle out"=w241:refnum<k15>)  [unwired: 7 in]
                n88 = call <instrlib>:"C63800 Set Fall Slew Rate of CR.vi"("error in (no error)"=w248, "Fall Slew Rate of CR"=w242, "Instrument Handle"=w241) -> ("error out"=w261:errorcluster)  [unwired: 7 in, 1 out]
              }
              frame "Rectified Mode (DC)" {
                w275 = T8 [enum."Current", enum."Current Peak", enum."Current Limit", enum."Crest Factor", enum."Frequency"] items=["Power", "Power Limit", "Current", "Current Peak", "Current Limit", "Voltage", "AC Resistance", "DC Resistance", "Frequency", "Crest Factor", "Power Factor", "RLC Power Factor", "Rise Slew Rate", "Fall Slew Rate", "Capacitance", "Inductance", "Parallel Resistance", "Series Resistance"] ("RangeCheck")
                w282 = 7 items=["CC", "CP", "CV", "CR", "RLC", "RLCP", "INRUSH", "RECT"] ("Load Mode")
                n89 = call-dynamic "CheckSettings.vi"("ChromaAcLoad in"=w276, "RangeCheck"=w275, "error in (no error)"=w278) -> ("error out"=w277:errorcluster)  [unwired: 6 in, 1 out]
                n90 = Unbundle By Name(w285) -> ("Synch Frequency (Hz)"=w264:dbl, "Crest Factor"=w274:dbl, "Load Current (A/Arms)"=w284:dbl, "Load Current Limit (A/Arms)"=w262:dbl, "Load Current Peak Limit (A)"=w263:dbl, "Line Synchronization"=w265:bool)
                n91 = call <instrlib>:"C63800 Set Load Mode.vi"("error in (no error)"=w277, "Load Mode"=w282, "Instrument Handle"=w279) -> ("error out"=w281:errorcluster, "Instrument Handle out"=w280:refnum<k15>)  [unwired: 7 in]
                n92 = call <instrlib>:"C63800 Set AC or DC Mode.vi"("error in (no error)"=w281, "Select AC_DC Mode"=TRUE, "Instrument Handle"=w280) -> ("error out"=w273:errorcluster, "Instrument Handle out"=w271:refnum<k15>)  [unwired: 7 in]
                n93 = call <instrlib>:"C63800 Set SYNC State of DC Rectified.vi"("error in (no error)"=w273, "SYNC State of DC Rectified"=w265, "Instrument Handle"=w271) -> ("error out"=w272:errorcluster, "Instrument Handle out"=w270:refnum<k15>)  [unwired: 7 in]
                n94 = call <instrlib>:"C63800 Set Ip(max) of DC.vi"("error in (no error)"=w272, "I_max_DC"=w263, "Instrument Handle"=w270) -> ("error out"=w267:errorcluster, "Instrument Handle out"=w266:refnum<k15>)  [unwired: 7 in]
                n95 = call <instrlib>:"C63800 Set Maximum RMS Current.vi"("error in (no error)"=w267, "Set Max RMS Current"=w262, "Instrument Handle"=w266) -> ("error out"=w269:errorcluster, "Instrument Handle out"=w268:refnum<k15>)  [unwired: 7 in]
                n96 = call <instrlib>:"C63800 Set RMS Current.vi"("error in (no error)"=w269, "Set RMS Current"=w284, "Instrument Handle"=w268) -> ("error out"=w290:errorcluster, "Instrument Handle out"=w289:refnum<k15>)  [unwired: 7 in]
                n97 = disable-structure shown="Disabled" {
                  disable-tunnel: w290 -> [w295 w296]
                  disable-tunnel: w289 -> [w294 w297]
                  disable-tunnel: [w293 w297] -> w288
                  disable-tunnel: [w292 w296] -> w287
                  disable-tunnel: w274 -> [w291 _]
                  frame Disabled {
                    n98 = call <instrlib>:"C63800 Set CF of DC.vi"("error in (no error)"=w295, "CF of DC"=w291, "Instrument Handle"=w294) -> ("error out"=w292:errorcluster, "Instrument Handle out"=w293:refnum<k15>)  [unwired: 7 in]
                  }
                  frame Enabled {
                  }
                }
                n99 = case shown="False" w265 {
                  tunnel: w288 -> [w301 _]
                  tunnel: w287 -> [w300 w302]
                  tunnel: [w299 w302] -> w286
                  tunnel: w264 -> [w298 _]
                  frame False {
                    n100 = call <instrlib>:"C63800 Set Frequency of DC Rectified.vi"("error in (no error)"=w300, "Frequency of DC Rectified"=w298, "Instrument Handle"=w301) -> ("error out"=w299:errorcluster)  [unwired: 7 in, 1 out]
                  }
                  frame True {
                  }
                }
              }
              frame "Inrush (AC)" {
                w312 = T8 [enum."Current", enum."Current Peak", enum."Current Limit", enum."Capacitance", enum."Inductance", enum."Current", enum."Parallel Resistance", enum."Series Resistance"] items=["Power", "Power Limit", "Current", "Current Peak", "Current Limit", "Voltage", "AC Resistance", "DC Resistance", "Frequency", "Crest Factor", "Power Factor", "RLC Power Factor", "Rise Slew Rate", "Fall Slew Rate", "Capacitance", "Inductance", "Parallel Resistance", "Series Resistance"] ("RangeCheck")
                w319 = 6 items=["CC", "CP", "CV", "CR", "RLC", "RLCP", "INRUSH", "RECT"] ("Load Mode")
                n101 = call-dynamic "CheckSettings.vi"("ChromaAcLoad in"=w315, "RangeCheck"=w312, "error in (no error)"=w314) -> ("error out"=w313:errorcluster)  [unwired: 6 in, 1 out]
                n102 = Unbundle By Name(w323) -> ("Load Current (A/Arms)"=w308:dbl, "LC/RLC Mode.Capacitance (uF)"=w328:i32, "LC/RLC Mode.Inductance (uH)"=w327:i32, "LC/RLC Mode.Parallel Resistance (Ohm)"=w326:dbl, "LC/RLC Mode.Series Resistance (Ohm)"=w325:dbl, "Load Current Limit (A/Arms)"=w303:dbl, "Load Current Peak Limit (A)"=w324:dbl)
                n103 = call <instrlib>:"C63800 Set Load Mode.vi"("error in (no error)"=w313, "Load Mode"=w319, "Instrument Handle"=w316) -> ("error out"=w318:errorcluster, "Instrument Handle out"=w317:refnum<k15>)  [unwired: 7 in]
                n104 = call <instrlib>:"C63800 Set AC or DC Mode.vi"("error in (no error)"=w318, "Select AC_DC Mode"=FALSE, "Instrument Handle"=w317) -> ("error out"=w322:errorcluster, "Instrument Handle out"=w321:refnum<k15>)  [unwired: 7 in]
                n105 = call <instrlib>:"C63800 Set Ip(max) of AC.vi"("error in (no error)"=w322, "Current Peak Max"=w324, "Instrument Handle"=w321) -> ("error out"=w305:errorcluster, "Instrument Handle out"=w304:refnum<k15>)  [unwired: 7 in]
                n106 = call <instrlib>:"C63800 Set Maximum RMS Current.vi"("error in (no error)"=w305, "Set Max RMS Current"=w303, "Instrument Handle"=w304) -> ("error out"=w307:errorcluster, "Instrument Handle out"=w306:refnum<k15>)  [unwired: 7 in]
                n107 = call <instrlib>:"C63800 Set RS of AC Inrush.vi"("error in (no error)"=w307, "RS of AC Inrush"=w325, "Instrument Handle"=w306) -> ("error out"=w330:errorcluster, "Instrument Handle out"=w329:refnum<k15>)  [unwired: 7 in]
                n108 = call <instrlib>:"C63800 Set RL of AC Inrush.vi"("error in (no error)"=w330, "RL of AC Inrush"=w326, "Instrument Handle"=w329) -> ("error out"=w334:errorcluster, "Instrument Handle out"=w333:refnum<k15>)  [unwired: 7 in]
                n109 = call <instrlib>:"C63800 Set LS of AC Inrush.vi"("error in (no error)"=w334, "LS of AC Inrush"=w327, "Instrument Handle"=w333) -> ("error out"=w332:errorcluster, "Instrument Handle out"=w331:refnum<k15>)  [unwired: 7 in]
                n110 = call <instrlib>:"C63800 Set C of AC Inrush.vi"("error in (no error)"=w332, "C of AC Inrush"=w328, "Instrument Handle"=w331) -> ("error out"=w311:errorcluster, "Instrument Handle out"=w309:refnum<k15>)  [unwired: 7 in]
                n111 = call <instrlib>:"C63800 Set RMS Current.vi"("error in (no error)"=w311, "Set RMS Current"=w308, "Instrument Handle"=w309) -> ("error out"=w310:errorcluster)  [unwired: 7 in, 1 out]
              }
              frame "RLC CP (AC)" {
                w344 = T8 [enum."Power", enum."Power Limit", enum."Current Peak", enum."RLC Power Factor"] items=["Power", "Power Limit", "Current", "Current Peak", "Current Limit", "Voltage", "AC Resistance", "DC Resistance", "Frequency", "Crest Factor", "Power Factor", "RLC Power Factor", "Rise Slew Rate", "Fall Slew Rate", "Capacitance", "Inductance", "Parallel Resistance", "Series Resistance"] ("RangeCheck")
                w351 = 5 items=["CC", "CP", "CV", "CR", "RLC", "RLCP", "INRUSH", "RECT"] ("Load Mode")
                n112 = Unbundle By Name(w356) -> ("Power Factor"=w341:dbl, "Load Power (W)"=w357:dbl, "Load Power Limit (W)"=w335:dbl, "Load Current Peak Limit (A)"=w355:dbl)
                n113 = call-dynamic "CheckSettings.vi"("ChromaAcLoad in"=w345, "RangeCheck"=w344, "error in (no error)"=w347) -> ("error out"=w346:errorcluster)  [unwired: 6 in, 1 out]
                n114 = call <instrlib>:"C63800 Set Load Mode.vi"("error in (no error)"=w346, "Load Mode"=w351, "Instrument Handle"=w349) -> ("error out"=w350:errorcluster, "Instrument Handle out"=w348:refnum<k15>)  [unwired: 7 in]
                n115 = call <instrlib>:"C63800 Set AC or DC Mode.vi"("error in (no error)"=w350, "Select AC_DC Mode"=FALSE, "Instrument Handle"=w348) -> ("error out"=w354:errorcluster, "Instrument Handle out"=w353:refnum<k15>)  [unwired: 7 in]
                n116 = call <instrlib>:"C63800 Set Ip(max) of AC.vi"("error in (no error)"=w354, "Current Peak Max"=w355, "Instrument Handle"=w353) -> ("error out"=w336:errorcluster, "Instrument Handle out"=w337:refnum<k15>)  [unwired: 7 in]
                n117 = call <instrlib>:"C63800 Set Maximum AC Power Loading.vi"("error in (no error)"=w336, "AC Maximum Power Loading"=w335, "Instrument Handle"=w337) -> ("error out"=w339:errorcluster, "Instrument Handle out"=w338:refnum<k15>)  [unwired: 7 in]
                n118 = call <instrlib>:"C63800 Set Power of AC RLC.vi"("error in (no error)"=w339, "Power of RLC"=w357, "Instrument Handle"=w338) -> ("error out"=w343:errorcluster, "Instrument Handle out"=w340:refnum<k15>)  [unwired: 7 in]
                n119 = call <instrlib>:"C63800 Set PF of AC RLC.vi"("error in (no error)"=w343, "PF of RLC"=w341, "Instrument Handle"=w340) -> ("error out"=w342:errorcluster)  [unwired: 7 in, 1 out]
              }
              frame "RLC (AC)" {
                w367 = T8 [enum."Current", enum."Current Peak", enum."Current Limit", enum."Capacitance", enum."Inductance", enum."Parallel Resistance", enum."Series Resistance"] items=["Power", "Power Limit", "Current", "Current Peak", "Current Limit", "Voltage", "AC Resistance", "DC Resistance", "Frequency", "Crest Factor", "Power Factor", "RLC Power Factor", "Rise Slew Rate", "Fall Slew Rate", "Capacitance", "Inductance", "Parallel Resistance", "Series Resistance"] ("RangeCheck")
                w375 = 4 items=["CC", "CP", "CV", "CR", "RLC", "RLCP", "INRUSH", "RECT"] ("Load Mode")
                n120 = call-dynamic "CheckSettings.vi"("ChromaAcLoad in"=w368, "RangeCheck"=w367, "error in (no error)"=w371) -> ("error out"=w370:errorcluster)  [unwired: 6 in, 1 out]
                n121 = call <instrlib>:"C63800 Set Load Mode.vi"("error in (no error)"=w370, "Load Mode"=w375, "Instrument Handle"=w373) -> ("error out"=w374:errorcluster, "Instrument Handle out"=w372:refnum<k15>)  [unwired: 7 in]
                n122 = Unbundle By Name(w378) -> ("Load Current (A/Arms)"=w363:dbl, "LC/RLC Mode.Capacitance (uF)"=w389:i32, "LC/RLC Mode.Inductance (uH)"=w386:i32, "LC/RLC Mode.Parallel Resistance (Ohm)"=w381:dbl, "LC/RLC Mode.Series Resistance (Ohm)"=w380:dbl, "Load Current Limit (A/Arms)"=w358:dbl, "Load Current Peak Limit (A)"=w379:dbl)
                n123 = call <instrlib>:"C63800 Set AC or DC Mode.vi"("error in (no error)"=w374, "Select AC_DC Mode"=FALSE, "Instrument Handle"=w372) -> ("error out"=w369:errorcluster, "Instrument Handle out"=w377:refnum<k15>)  [unwired: 7 in]
                n124 = call <instrlib>:"C63800 Set Ip(max) of AC.vi"("error in (no error)"=w369, "Current Peak Max"=w379, "Instrument Handle"=w377) -> ("error out"=w362:errorcluster, "Instrument Handle out"=w361:refnum<k15>)  [unwired: 7 in]
                n125 = call <instrlib>:"C63800 Set Maximum RMS Current.vi"("error in (no error)"=w362, "Set Max RMS Current"=w358, "Instrument Handle"=w361) -> ("error out"=w360:errorcluster, "Instrument Handle out"=w359:refnum<k15>)  [unwired: 7 in]
                n126 = call <instrlib>:"C63800 Set RS of AC RLC.vi"("error in (no error)"=w360, "RS of RLC"=w380, "Instrument Handle"=w359) -> ("error out"=w383:errorcluster, "Instrument Handle out"=w382:refnum<k15>)  [unwired: 7 in]
                n127 = call <instrlib>:"C63800 Set RL of AC RLC.vi"("error in (no error)"=w383, "RL of RLC"=w381, "Instrument Handle"=w382) -> ("error out"=w384:errorcluster, "Instrument Handle out"=w385:refnum<k15>)  [unwired: 7 in]
                n128 = call <instrlib>:"C63800 Set Ls of AC RLC.vi"("error in (no error)"=w384, "Ls of RLC"=w386, "Instrument Handle"=w385) -> ("error out"=w388:errorcluster, "Instrument Handle out"=w387:refnum<k15>)  [unwired: 7 in]
                n129 = call <instrlib>:"C63800 Set C of AC RLC.vi"("error in (no error)"=w388, "The Value C"=w389, "Instrument Handle"=w387) -> ("error out"=w366:errorcluster, "Instrument Handle out"=w365:refnum<k15>)  [unwired: 7 in]
                n130 = call <instrlib>:"C63800 Set RMS Current.vi"("error in (no error)"=w366, "Set RMS Current"=w363, "Instrument Handle"=w365) -> ("error out"=w364:errorcluster)  [unwired: 7 in, 1 out]
              }
            }
          }
        }
      }
    }
    frame Error {
    }
  }
  "error out" <- w6
  "ChromaAcLoad out" <- w5
